vi "subDescendentsToLinkerLibs.vi"(7 "Build spec override":string, 9 "All descendents":refnum<vi>[](array[refnum]), 10 "Name":string, 11 "Map in":map{string, set{string}}(c390)) -> (3 "Map out":map{string, set{string}}(c390))   [LabVIEW 2020, in "SolutionBuilder.lvlib" / "SolutionBuilder.lvclass"]
uses:
  SolutionBuilder.lvclass
  <vilib>/Utility/miscctls.llb/LVMapReplaceAction.ctl
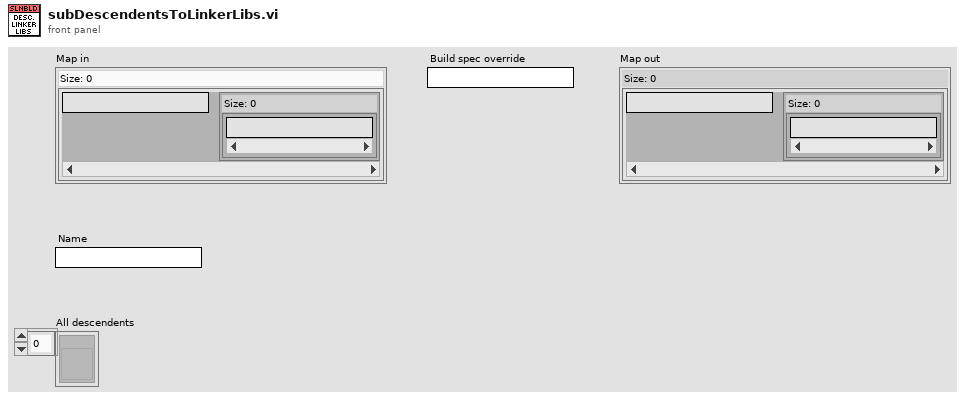
[diagram p1: front panel]
types:
  T1 = typedef "LVMapReplaceAction.ctl" = enum32{"Modify Entry only if found", "Add or Modify Entry", "Delete Entry"}
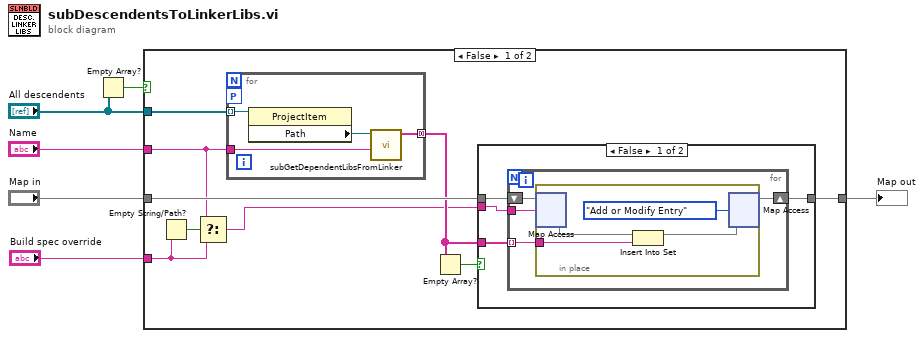
[diagram p0: block diagram]
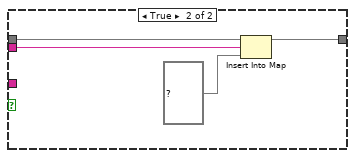
[diagram p2: hidden frame]
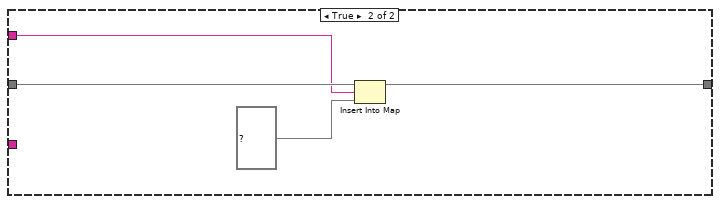
[diagram p3: hidden frame]
diagram:
  n1 = Empty Array?(array="All descendents") -> (empty?=w6:bool)
  n2 = case shown="False" w6 {
    tunnel: "Map in" -> [w15 w39]
    tunnel: [w14 w38] -> w3
    tunnel: "All descendents" -> [w13 _]
    tunnel: "Name" -> [w8 w36]
    tunnel: "Build spec override" -> [w9 _]
    frame False {
      n3 = Empty String/Path?(string/path=w9) -> (empty?=w10:bool)
      n4 = Select(t=w8, s=w10, f=w9) -> (s? t:f=w7:string)
      n5 = for {
        tunnel: w13 -> [w19] mode=indexing
        workers-P: _ -> [_]
        tunnel: [w17] -> w12 mode=concatenating
        tunnel: w8 -> [w16]
        n6 = property class="ProjectItem"(reference=w19) -> ("Path"=w18:path)  [unwired: 1 in, 2 out]
        n7 = call "subGetDependentLibsFromLinker.vi"("Name"=w16, "Path"=w18) -> ("Dependent libs"=w17:string[])  [unwired: 9 in]
      }
      n8 = Empty Array?(array=w12) -> (empty?=w11:bool)
      n9 = case shown="False" w11 {
        tunnel: w15 -> [w23 w34]
        tunnel: [w22 w33] -> w14
        tunnel: w7 -> [w21 w32]
        tunnel: w12 -> [w20 _]
        frame False {
          n10 = for {
            shift-right: [w26] -> w22
            shift-left: w23 -> [w27]
            tunnel: w21 -> [w25]
            tunnel: w20 -> [w24] mode=indexing
            n11 = in-place {
              in-place-border: w24 -> [w30]
              n12 = in-place-map #1(w27, w25) -> (w31:set{string})  [unwired: 1 in, 1 out]
              n13 = Insert Into Set(10:w30, 11:w31) -> (3:w29:set{string})  [unwired: 1 out]
              n14 = in-place-map #1(w29, LVMapReplaceAction."Add or Modify Entry" ("action")) -> (w26:map{string, set{string}})  [unwired: 2 out]
            }
          }
        }
        frame True {
          n15 = Insert Into Map(map in=w34, key=w32, value=set{string} {}) -> (map out=w33:map{string, set{string}})  [unwired: 2 out]
        }
      }
    }
    frame True {
      n16 = Insert Into Map(map in=w39, key=w36, value=set{string} {}) -> (map out=w38:map{string, set{string}})  [unwired: 2 out]
    }
  }
  "Map out" <- w3
